vi "Servo Tracking State Machine.vi"(0 "Servo Positions In":cluster{"X":dbl, "Y":dbl}, 1 "Image Size":T4=enum."320x240", 7 "Rectangle":T3, 9 "Particles":i32, 11 "Area":i32=4, 12 "Left?":bool=TRUE, 13 "Center":cluster{"X":dbl, "Y":dbl}) -> (4 "Servo Positions":cluster{"X":dbl, "Y":dbl}, 6 "Tracking State Info":T2)   [LabVIEW 2013]
uses:
  Control States.ctl
  <vilib>/Rock Robotics/WPI/Camera/WPI_CameraImageSize.ctl
panel:
  in  "Upper Limit":cluster{"X":i32, "Y":i32}={"X"=169, "Y"=130}
  in  "Lower Limit":cluster{"X":i32, "Y":i32}={"X"=0, "Y"=40}
  in  "Search Speed":i32=4
  in  "Proportional (div)":cluster{"X":i32, "Y":i32}={"X"=15, "Y"=-13}
  # "Unwired tuning params for control.\nSearch speed determines how fast the\ngimbal will move when trying to acquire\na target. Too fast and you may miss the\ntarget between frames, too slow is boring.\n\nProportional(div) is the proportional constant\nexpressed as a divisor term. Adjust this higher\nif the gimbal is oscillating, lower for quicker\nresponse.\n\nThe limits are useful for keeping the gimbal in\na working range, some stick when the get near\ntheir mechanical limits. It is also useful to limit\nthe searching to avoid looking at the ceiling, etc."
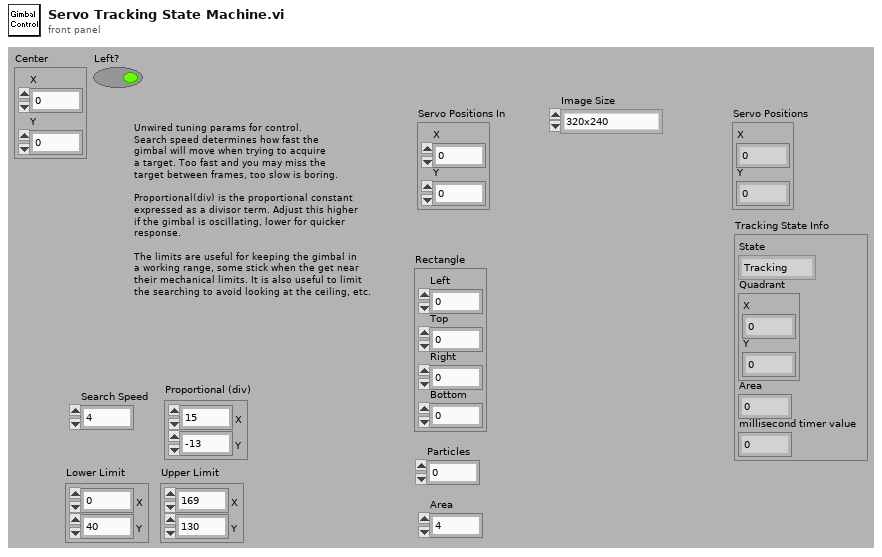
[diagram p1: front panel]
types:
  T1 = typedef "Control States.ctl" = enum16{"Tracking", "Lost Small", "Lost-Patience", "Search-Begin", "Searching", "Lost - Edge"}
  T2 = cluster{"State":T1, "Quadrant":cluster{"X":i32, "Y":i32}, "Area":i32, "millisecond timer value":u32}
  T3 = cluster{"Left":i32, "Top":i32, "Right":i32, "Bottom":i32}
  T4 = typedef "WPI_CameraImageSize.ctl" = enum16{"640x480", "320x240", "160x120"}
  T5 = cluster{"State":T1, "Grid Element":cluster{"X":i32, "Y":i32}, "Area":i32, "millisecond timer value":u32}
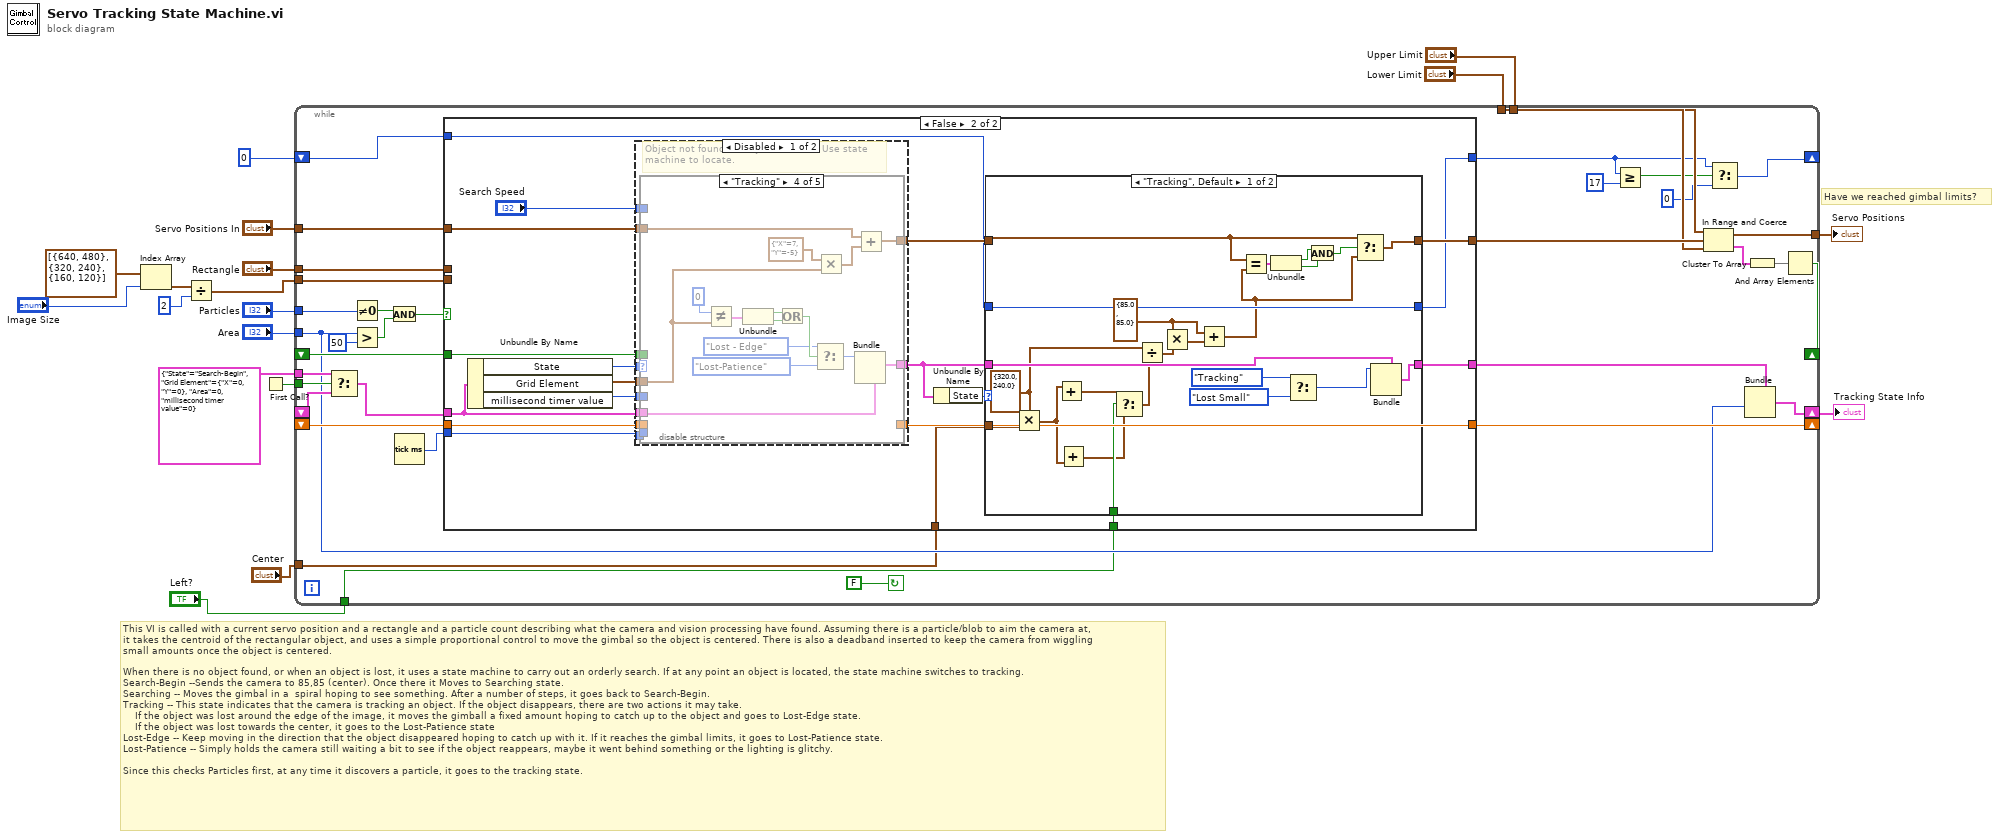
[diagram p0: block diagram]
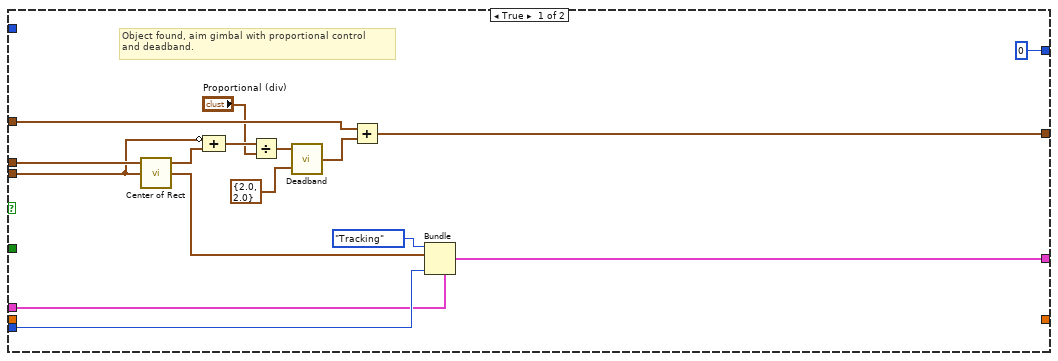
[diagram p2: hidden frame]
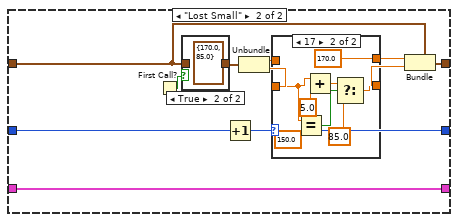
[diagram p3: hidden frame]
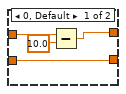
[diagram p4: hidden frame]
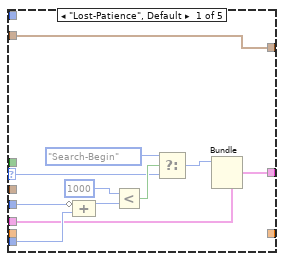
[diagram p6: hidden frame]
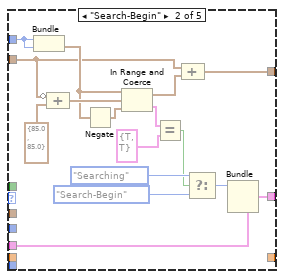
[diagram p7: hidden frame]
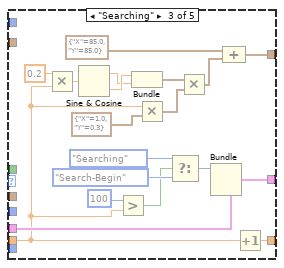
[diagram p8: hidden frame]
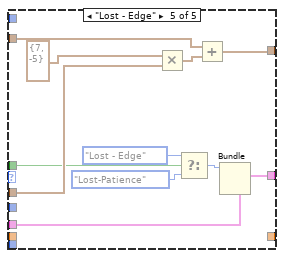
[diagram p9: hidden frame]
diagram:
  # "Have we reached gimbal limits?"
  # "This VI is called with a current servo position and a rectangle and a particle count describing what the camera and vision processing have found. Assuming there is a particle/blob to aim the camera at,\nit takes the centroid of the rectangular object, and uses a simple proportional control to move the gimbal so the object is centered. There is also a deadband inserted to keep the camera from wiggling\nsmall amounts once the object is centered.\n\nWhen there is no object found, or when an object is lost, it uses a state machine to carry out an orderly search. If at any point an object is located, the state machine switches to tracking.\nSearch-Begin --Sends the camera to 85,85 (center). Once there it Moves to Searching state.\nSearching -- Moves the gimbal in a  spiral hoping to see something. After a number of steps, it goes back to Search-Begin.\nTracking -- This state indicates that the camera is tracking an object. If the object disappears, there are two actions it may take.\n    If the object was lost around the edge of the image, it moves the gimball a fixed amount hoping to catch up to the object and goes to Lost-Edge state.\n    If the object was lost towards the center, it goes to the Lost-Patience state\nLost-Edge -- Keep moving in the direction that the object disappeared hoping to catch up with it. If it reaches the gimbal limits, it goes to Lost-Patience state.\nLost-Patience -- Simply holds the camera still waiting a bit to see if the object reappears, maybe it went behind something or the lighting is glitchy.\n\nSince this checks Particles first, at any time it discovers a particle, it goes to the tracking state."
  n1 = Index Array(array=cluster{"X":i32, "Y":i32}[] [{"X"=640, "Y"=480}, {"X"=320, "Y"=240}, {"X"=160, "Y"=120}] ("Resolutions"), index="Image Size") -> (element=w15:cluster{"X":i32, "Y":i32})
  n2 = Divide(x=w15, y=2) -> (x/y=w16:cluster{"X":dbl, "Y":dbl})
  n3 = First Call?() -> (First Call?: T/F=w8:bool)
  n4 = while {
    tunnel: w16 -> [w35]
    tunnel: "Particles" -> [w34]
    tunnel: "Rectangle" -> [w36]
    tunnel: [w44] -> w11
    shift-right: [w52] -> _
    shift-left: _ -> [w51]
    tunnel: "Servo Positions In" -> [w50]
    shift-right: [w29] -> w9
    shift-left: _ -> [w47]
    tunnel: w8 -> [w49]
    tunnel: T5 {"State"=enum."Search-Begin", "Grid Element"={"X"=0, "Y"=0}, "Area"=0, "millisecond timer value"=0} -> [w48]
    tunnel: "Lower Limit" -> [w42]
    tunnel: "Upper Limit" -> [w41]
    shift-right: [w38] -> _
    shift-left: _ -> [w37]
    tunnel: "Area" -> [w27]
    shift-right: [w25] -> _
    shift-left: 0 -> [w26]
    tunnel: "Center" -> [w20]
    tunnel: "Left?" -> [w19]
    stop <- FALSE continue-if-true
    n5 = Select(t=w48, s=w49, f=w47) -> (s? t:f=w46:T5)
    n6 = Not Equal To 0?(x=w34) -> (x != 0?=w32:bool)
    n7 = Greater?(x=w27, y=50) -> (0:w31:bool)
    n8 = And(x=w32, y=w31) -> (x .and. y?=w30:bool)
    n9 = Tick Count (ms)() -> (millisecond timer value=w53:u32)
    n10 = case shown="False" w30 {
      tunnel: w36 -> [w58 _]
      tunnel: w35 -> [w55 _]
      tunnel: w53 -> [w65 w88]
      tunnel: [w67 w73] -> w28
      tunnel: w46 -> [w59 w82]
      tunnel: w50 -> [w66 w87]
      tunnel: [w64 w76] -> w43
      tunnel: w51 -> [_ w86]
      tunnel: [_ w85] -> w52
      tunnel: w37 -> [_ w84]
      tunnel: w26 -> [_ w75]
      tunnel: [0 w74] -> w24
      tunnel: w20 -> [_ w71]
      tunnel: w19 -> [_ w70]
      frame True {
        # "Object found, aim gimbal with proportional control\nand deadband."
        n11 = call "Center of Rect.vi"("Camera Center"=w55, "Rectangle"=w58) -> ("Grid Element"=w56:cluster{"X":i32, "Y":i32}, "Center"=w57:cluster{dbl, dbl})  [unwired: 1 in, 1 out]
        n12 = Compound Arithmetic op=ADD(invert w55, w57) -> (w69:cluster{dbl, dbl})
        n13 = Divide(x=w69, y="Proportional (div)") -> (x/y=w62:cluster{dbl, dbl})
        n14 = call "Deadband.vi"("Deadband"=cluster{dbl, dbl} {2.0, 2.0}, "Value"=w62) -> ("Value Out"=w61:cluster{dbl, dbl})
        n15 = Add(x=w66, y=w61) -> (x+y=w64:cluster{dbl, dbl})
        n16 = Bundle(cluster=w59, "State"=Control_States."Tracking", "Grid Element"=w56, "millisecond timer value"=w65) -> (w67:T5)  [unwired: 1 out]
      }
      frame False {
        n17 = Unbundle By Name(w82) -> ("State"=w81:T1, "Grid Element"=w80:cluster{"X":i32, "Y":i32}, "millisecond timer value"=w79:u32)
        n18 = disable-structure shown="Disabled" {
          disable-tunnel: [w148 _] -> w72
          disable-tunnel: w88 -> [w147 _]
          disable-tunnel: [w146 _] -> w77
          disable-tunnel: w87 -> [w145 _]
          disable-tunnel: w86 -> [w144 _]
          disable-tunnel: [w143 _] -> w85
          disable-tunnel: w84 -> [w142 _]
          disable-tunnel: "Search Speed" -> [w141 _]
          disable-tunnel: w82 -> [w140 _]
          disable-tunnel: w81 -> [w139 _]
          disable-tunnel: w80 -> [w138 _]
          disable-tunnel: w79 -> [w137 _]
          frame Disabled {
            # "Object not found, or object was lost. Use state\nmachine to locate."
            n19 = case shown="\"Tracking\"" w139 {
              selector: w139 -> [w150 _ _ _ _]
              tunnel: [w151 w166 w181 w209 w220] -> w148
              tunnel: w140 -> [w155 w167 w182 w208 w219]
              tunnel: w137 -> [w158 _ _ _ _]
              tunnel: w147 -> [w159 _ _ _ _]
              tunnel: [w149 w168 w186 w200 w215] -> w146
              tunnel: w145 -> [w149 w169 _ w199 w216]
              tunnel: w141 -> [_ w173 _ _ _]
              tunnel: w144 -> [_ _ w177 _ _]
              tunnel: [_ _ w194 _ _] -> w143
              tunnel: w138 -> [_ _ _ w196 w214]
              tunnel: w142 -> [_ _ _ _ w210]
              frame "Lost-Patience", Default {
                n20 = Compound Arithmetic op=ADD(invert w158, w159) -> (w157:u32)
                n21 = Less?(x=1000, y=w157) -> (x < y?=w152:bool)
                n22 = Select(t=Control_States."Search-Begin" ("State"), s=w152, f=w150) -> (s? t:f=w154:T1)
                n23 = Bundle(cluster=w155, "State"=w154) -> (w151:T5)  [unwired: 3 out]
              }
              frame "Search-Begin" {
                n24 = Bundle("Search Speed"=w173, "Search Speed"=w173) -> (w172:cluster{"Search Speed":i32, "Search Speed":i32})  [unwired: 1 out]
                n25 = Compound Arithmetic op=ADD(invert w169, cluster{"X":dbl, "Y":dbl} {"X"=85.0, "Y"=85.0} ("Servos")) -> (w174:cluster{"X":dbl, "Y":dbl})
                n26 = Negate(x=w172) -> (-x=w171:cluster{"Search Speed":i32, "Search Speed":i32})
                n27 = In Range and Coerce(upper limit=w172, x=w174, lower limit=w171) -> (coerced(x)=w170:cluster{"X":dbl, "Y":dbl}, In Range?=w162:cluster{"X":bool, "Y":bool})
                n28 = Equal?(x=w162, y=cluster{"X":bool, "Y":bool} {"X"=TRUE, "Y"=TRUE}) -> (x = y?=w160:bool)
                n29 = Compound Arithmetic op=ADD(w169, w170) -> (w168:cluster{"X":dbl, "Y":dbl})
                n30 = Select(t=Control_States."Searching" ("State"), s=w160, f=Control_States."Search-Begin" ("State")) -> (s? t:f=w165:T1)
                n31 = Bundle(cluster=w167, "State"=w165) -> (w166:T5)  [unwired: 3 out]
              }
              frame "Searching" {
                n32 = Multiply(x=0.2, y=w177) -> (x*y=w192:dbl)
                n33 = Sine & Cosine(0:w192) -> (1:w190:dbl, 2:w191:dbl)
                n34 = Greater?(x=100, y=w177) -> (0:w179:bool)
                n35 = Bundle(w191, w190) -> (w189:cluster{dbl, dbl})  [unwired: 1 out]
                n36 = Multiply(x=w177, y=cluster{"X":dbl, "Y":dbl} {"X"=1.0, "Y"=0.3} ("Servos")) -> (x*y=w178:cluster{"X":dbl, "Y":dbl})
                n37 = Select(t=Control_States."Searching" ("State"), s=w179, f=Control_States."Search-Begin" ("State")) -> (s? t:f=w185:T1)
                n38 = Multiply(x=w189, y=w178) -> (x*y=w188:cluster{dbl, dbl})
                n39 = Bundle(cluster=w182, "State"=w185) -> (w181:T5)  [unwired: 3 out]
                n40 = Compound Arithmetic op=ADD(cluster{"X":dbl, "Y":dbl} {"X"=85.0, "Y"=85.0} ("Servos"), w188) -> (w186:cluster{dbl, dbl})
                n41 = Increment(x=w177) -> (x+1=w194:dbl)
              }
              frame "Tracking" {
                n42 = Not Equal?(x=0 ("X"), y=w196) -> (x != y?=w207:cluster{"X":bool, "Y":bool})
                n43 = Unbundle(w207) -> ("X"=w206:bool, "Y"=w205:bool)
                n44 = Or(x=w206, y=w205) -> (x .or. y?=w204:bool)
                n45 = Select(t=Control_States."Lost - Edge" ("State"), s=w204, f=Control_States."Lost-Patience" ("State")) -> (s? t:f=w201:T1)
                n46 = Multiply(x=cluster{"X":i32, "Y":i32} {"X"=7, "Y"=-5}, y=w196) -> (x*y=w198:cluster{"X":i32, "Y":i32})
                n47 = Bundle(cluster=w208, "State"=w201) -> (w209:T5)  [unwired: 3 out]
                n48 = Add(x=w199, y=w198) -> (x+y=w200:cluster{"X":dbl, "Y":dbl})
              }
              frame "Lost - Edge" {
                n49 = Multiply(x=cluster{"X":i32, "Y":i32} {"X"=7, "Y"=-5}, y=w214) -> (x*y=w218:cluster{"X":i32, "Y":i32})
                n50 = Select(t=Control_States."Lost - Edge" ("State"), s=w210, f=Control_States."Lost-Patience" ("State")) -> (s? t:f=w213:T1)
                n51 = Add(x=w216, y=w218) -> (x+y=w215:cluster{"X":dbl, "Y":dbl})
                n52 = Bundle(cluster=w219, "State"=w213) -> (w220:T5)  [unwired: 3 out]
              }
            }
          }
          frame Enabled {
          }
        }
        n53 = Unbundle By Name(w72) -> ("State"=w78:T1)
        n54 = case shown="\"Tracking\", Default" w78 {
          tunnel: w77 -> [w107 w119]
          tunnel: [w108 w120] -> w76
          tunnel: w75 -> [w111 w113]
          tunnel: [w111 w113] -> w74
          tunnel: [w110 w112] -> w73
          tunnel: w72 -> [w109 w112]
          tunnel: w71 -> [w99 _]
          tunnel: w70 -> [w101 _]
          frame "Tracking", Default {
            w92 = cluster{"X":dbl, "Y":dbl} {"X"=85.0, "Y"=85.0} ("x")
            w95 = cluster{"X":dbl, "Y":dbl} {"X"=320.0, "Y"=240.0} ("x")
            n55 = Multiply(x=w95, y=w99) -> (x*y=w98:cluster{"X":dbl, "Y":dbl})
            n56 = Add(x=w98) -> (x+y=w102:cluster{"X":dbl, "Y":dbl})  [unwired: 1 in]
            n57 = Add(y=w98) -> (x+y=w100:cluster{"X":dbl, "Y":dbl})  [unwired: 1 in]
            n58 = Select(t=w102, s=w101, f=w100) -> (s? t:f=w96:cluster{"X":dbl, "Y":dbl})
            n59 = Divide(x=w95, y=w96) -> (x/y=w97:cluster{"X":dbl, "Y":dbl})
            n60 = Multiply(x=w92, y=w97) -> (x*y=w93:cluster{"X":dbl, "Y":dbl})
            n61 = Add(x=w92, y=w93) -> (x+y=w94:cluster{"X":dbl, "Y":dbl})
            n62 = Equal?(x=w107, y=w94) -> (x = y?=w105:cluster{"X":bool, "Y":bool})
            n63 = Unbundle(w105) -> ("X"=w104:bool, "Y"=w103:bool)
            n64 = Select(t=Control_States."Tracking" ("State"), f=Control_States."Lost Small") -> (s? t:f=w90:T1)  [unwired: 1 in]
            n65 = And(x=w104, y=w103) -> (x .and. y?=w106:bool)
            n66 = Select(t=w107, s=w106, f=w94) -> (s? t:f=w108:cluster{"X":dbl, "Y":dbl})
            n67 = Bundle(cluster=w109, "State"=w90) -> (w110:T5)  [unwired: 3 in]
          }
          frame "Lost Small" {
            n68 = First Call?() -> (First Call?: T/F=w122:bool)
            n69 = case shown="True" w122 {
              tunnel: w119 -> [w135 _]
              tunnel: [w135 cluster{"X":dbl, "Y":dbl} {"X"=170.0, "Y"=85.0} ("Servo Positions In")] -> w121
              frame False {
              }
              frame True {
              }
            }
            n70 = Increment(x=w113) -> (x+1=w118:i32)
            n71 = Unbundle(w121) -> ("X"=w117:dbl, "Y"=w116:dbl)
            n72 = case shown="17" w118 {
              tunnel: w117 -> [w125 _]
              tunnel: w116 -> [w126 w128]
              tunnel: [w124 170.0] -> w115
              tunnel: [w126 w133] -> w114
              frame 0, Default {
                n73 = Subtract(x=w125, y=10.0) -> (x-y=w124:dbl)
              }
              frame 17 {
                n74 = Equal?(x=w128, y=150.0) -> (x = y?=w130:bool)
                n75 = Add(x=w128, y=5.0) -> (x+y=w132:dbl)
                n76 = Select(t=w132, s=w130, f=85.0) -> (s? t:f=w133:dbl)
              }
            }
            n77 = Bundle(cluster=w119, "X"=w115, "Y"=w114) -> (w120:cluster{"X":dbl, "Y":dbl})
          }
        }
      }
    }
    n78 = Greater Or Equal?(x=w24, y=17) -> (x >= y?=w22:bool)
    n79 = In Range and Coerce(upper limit=w41, x=w43, lower limit=w42) -> (coerced(x)=w44:cluster{"X":dbl, "Y":dbl}, In Range?=w40:cluster{"X":bool, "Y":bool})
    n80 = Select(t=w24, s=w22, f=0) -> (s? t:f=w25:i32)
    n81 = Bundle(cluster=w28, "Area"=w27) -> (w29:T5)  [unwired: 3 out]
    n82 = Cluster To Array(cluster=w40) -> (array=w39:bool[])
    n83 = And Array Elements(Boolean array=w39) -> (logical AND=w38:bool)
  }
  "Servo Positions" <- w11
  "Tracking State Info" <- w9
